vi "Dequeue Message.vi"(8 "error in (no error)":errorcluster, 11 "Message Queue in":refnum<queue>) -> (0 "error out":errorcluster, 1 "Data":variant, 2 "State":string, 3 "Message Queue out":refnum<queue>)   [LabVIEW 2016, in "Message Queue.lvlib"]
uses:
  Message Queue.lvlib
  Message.ctl
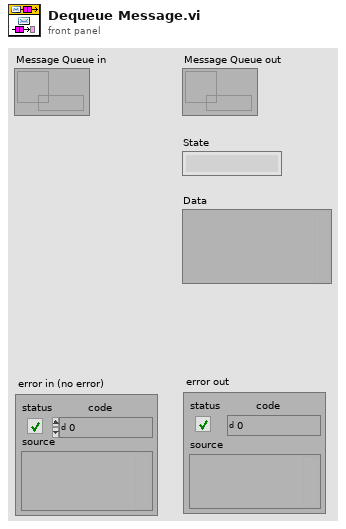
[diagram p1: front panel]
types:
  T1 = typedef "Message Queue.lvlib/Message.ctl" = cluster{"State":string, "Data":variant}
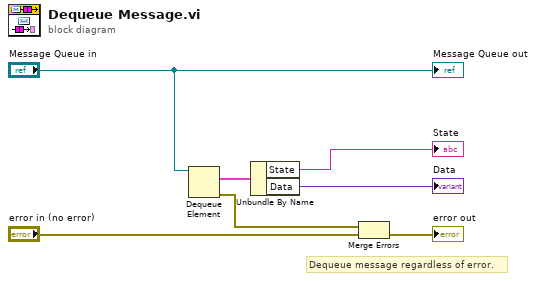
[diagram p0: block diagram]
diagram:
  # "Dequeue message regardless of error."
  n1 = Dequeue Element(queue="Message Queue in") -> (element=w3:T1, error out=w4:errorcluster)  [unwired: 2 in, 2 out]
  n2 = Unbundle By Name(w3) -> ("State"=→"State":string, "Data"=→"Data":variant)
  n3 = Merge Errors(w4, "error in (no error)") -> (→"error out":errorcluster)
  "Message Queue out" <- "Message Queue in"
